vi "VAT_valve_get_type.vi"(0 "VAT Valve COM port":refnum<visa-resource-name>, 11 "error in (no error)":errorcluster) -> (4 "VAT Valve COM port out":refnum<visa-resource-name>, 13 "Valve Type":string, 15 "error out":errorcluster)   [LabVIEW 2019]
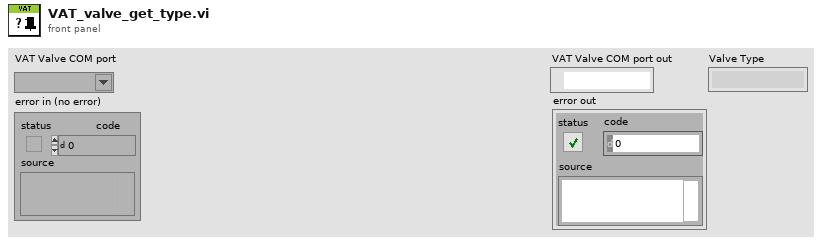
[diagram p1: front panel]
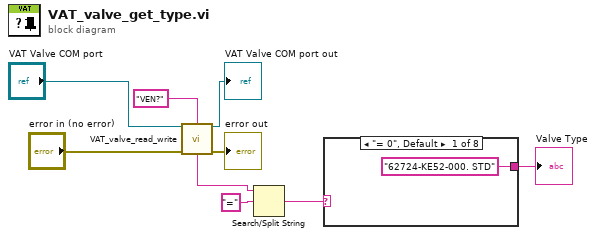
[diagram p0: block diagram]
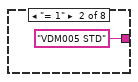
[diagram p2: hidden frame]
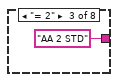
[diagram p3: hidden frame]
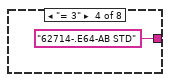
[diagram p4: hidden frame]
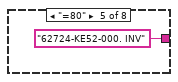
[diagram p5: hidden frame]
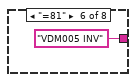
[diagram p6: hidden frame]
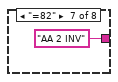
[diagram p7: hidden frame]
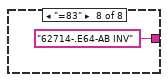
[diagram p8: hidden frame]
diagram:
  n1 = call "VAT_valve_read_write.vi"("VAT Valve COM port"="VAT Valve COM port", "Write String"="VEN?", "error in (no error)"="error in (no error)") -> ("VAT Valve COM port out"=→"VAT Valve COM port out":refnum<visa-resource-name>, "Read String"=w3:string, "error out"=→"error out":errorcluster)  [unwired: 10 in]
  n2 = Search/Split String(string=w3, search string/char (-)="=") -> (match + rest of string=w9:string)  [unwired: 1 in, 2 out]
  n3 = case shown="\"= 0\", Default" w9 {
    tunnel: ["62724-KE52-000. STD" "VDM005 STD" "AA 2 STD" "62714-.E64-AB STD" "62724-KE52-000. INV" "VDM005 INV" "AA 2 INV" "62714-.E64-AB INV"] -> w7
    frame "= 0", Default {
    }
    frame "= 1" {
    }
    frame "= 2" {
    }
    frame "= 3" {
    }
    frame "=80" {
    }
    frame "=81" {
    }
    frame "=82" {
    }
    frame "=83" {
    }
  }
  "Valve Type" <- w7
